vi "DBVar ClassificationDataInput.vi"(1 "data wired":bool, 2 "data":variant, 3 "old data classification":T1(ring)) -> (0 "data classification":T1(ring))   [LabVIEW 2012, in "NI_DB Variant To Data Support.lvlib"]
uses:
  NI_DB Variant To Data Support.lvlib
  <vilib>/Utility/VariantDataType/Type.ctl
  <vilib>/Utility/VariantDataType/VariantType.lvlib
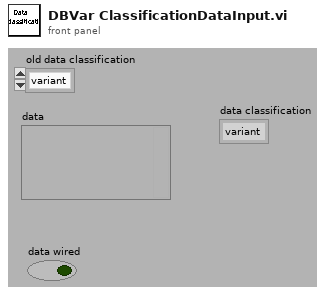
[diagram p1: front panel]
types:
  T1 = enum16{"variant", "variant 1D array", "variant 2D array", "others"}
  T2 = typedef "VariantType.lvlib/Type.ctl" = enum8{"Invalid Type", "Void", "I8", "I16", "I32", "I64", "U8", "U16", "U32", "U64", "Single Float", "Double Float", "Extended Float", "Single Complex", "Double Complex", "Extended Complex", "Enum U8", "Enum U16", "Enum U32", "Enum U64", "Single Float With Unit", "Double Float With Unit", "Extended Float With Unit", "Single Complex with Unit", "Double Complex with Unit", "Extended Complex with Unit", "Boolean", "String", "Path", "Picture", "Tag", "Array", "Cluster", "Variant", "LV Variant", "Waveform", "Timestamp", "Digital Waveform", "Digital Data", "ExpressData", "Refnum", "External Data", "VI", "Poly VI", "LabVIEW Class Instance", "Fixed Point"}
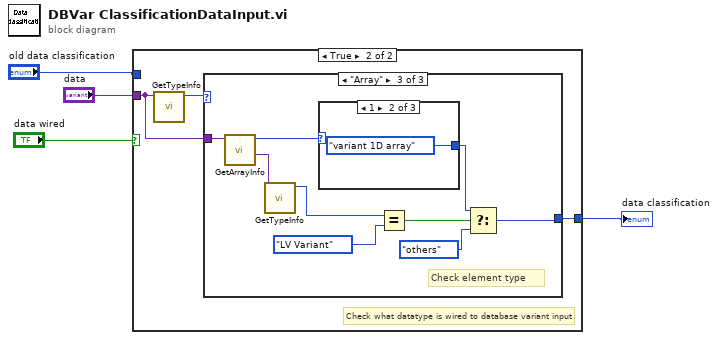
[diagram p0: block diagram]
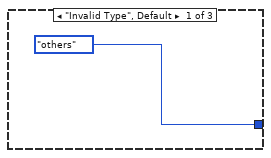
[diagram p3: hidden frame]
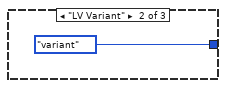
[diagram p4: hidden frame]
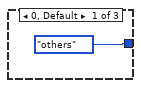
[diagram p5: hidden frame]
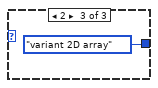
[diagram p6: hidden frame]
diagram:
  n1 = case shown="True" "data wired" {
    tunnel: "data" -> [_ w6]
    tunnel: [w5 w7] -> w4
    tunnel: "old data classification" -> [w5 _]
    frame False {
      # "Input not wired, do not change data input"
    }
    frame True {
      # "Check what datatype is wired to database variant input"
      n2 = call <vilib>:"GetTypeInfo.vi"("Variant"=w6) -> ("Type Enum"=w8:T2)  [unwired: 1 in, 9 out]
      n3 = case shown="\"Array\"" w8 {
        tunnel: [T1."others" ("data") T1."variant" ("data") w11] -> w7
        tunnel: w6 -> [_ _ w12]
        frame "Invalid Type", Default {
        }
        frame "LV Variant" {
        }
        frame "Array" {
          # "Check element type"
          n4 = call <vilib>:"GetArrayInfo.vi"("Variant"=w12) -> ("ArrayElement"=w19:variant, "NDims"=w16:i32)  [unwired: 7 in, 2 out]
          n5 = call <vilib>:"GetTypeInfo.vi"("Variant"=w19) -> ("Type Enum"=w14:T2)  [unwired: 1 in, 9 out]
          n6 = case shown="1" w16 {
            tunnel: [T1."others" ("data") T1."variant 1D array" ("data") T1."variant 2D array" ("data")] -> w13
            frame 0, Default {
            }
            frame 1 {
            }
            frame 2 {
            }
          }
          n7 = Equal?(x=w14, y=Type."LV Variant" ("Type Enum")) -> (x = y?=w18:bool)
          n8 = Select(t=w13, s=w18, f=T1."others" ("data")) -> (s? t:f=w11:T1)
        }
      }
    }
  }
  "data classification" <- w4
